vi "SAVEHWS.vi"(8 "error in (no error)":errorcluster, 9 "Enable (Array)":bool[](array[boolean]), 10 "data":waveform(dbl)[](array[waveform]), 11 "Destination HWS File":path) -> (0 "error out":errorcluster)   [LabVIEW 2011, in "DaqPad_NI6009.lvclass"]
uses:
  DaqPad_NI6009.lvclass
  niHWS Open File Permissions ID.ctl
panel:
  out "Waveform":waveform(dbl)(graph)
  out "Numeric":i32
  out "Array":string[](array[string])
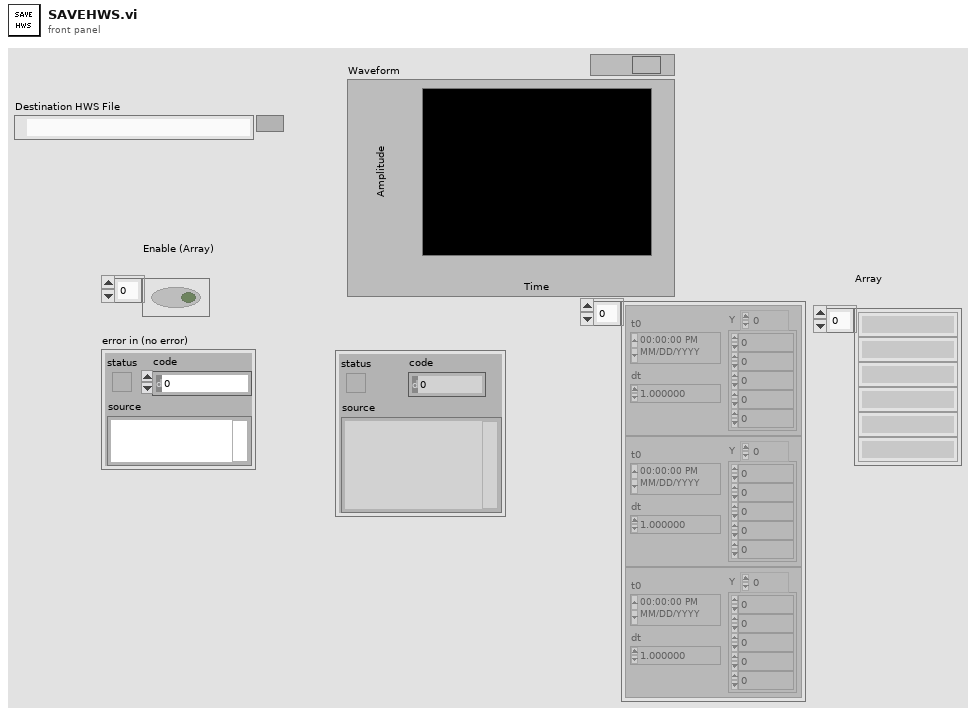
[diagram p1: front panel]
types:
  T1 = typedef "niHWS Open File Permissions ID.ctl" = enum32{"Read Only", "Read/Write Existing", "Read/Write/Create New", "Read/Write/Create New Always"}
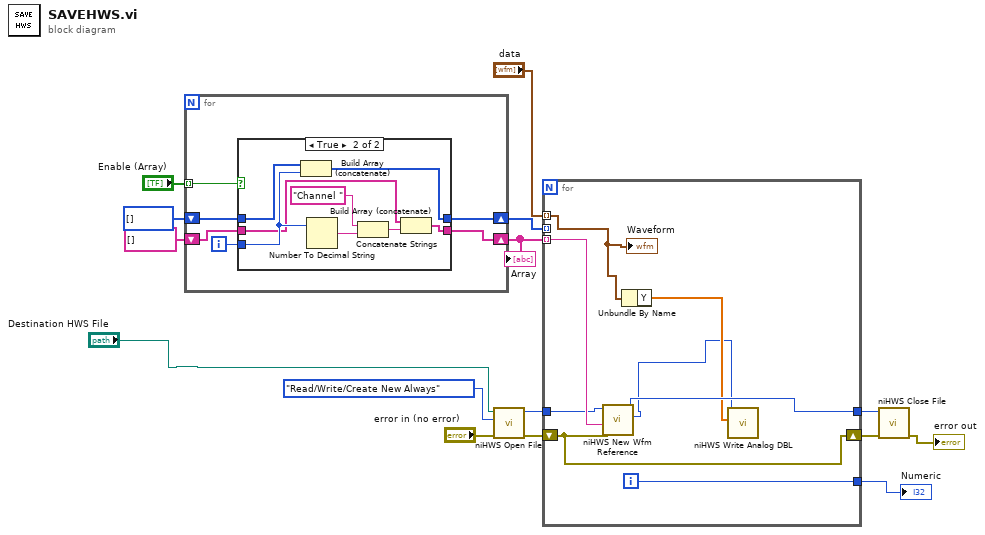
[diagram p0: block diagram]
diagram:
  n1 = for {
    tunnel: "Enable (Array)" -> [w21] mode=indexing
    shift-right: [w19] -> w14
    shift-left: i32[] [] -> [w18]
    shift-right: [w17] -> w15
    shift-left: string[] [] -> [w16]
    i -> [w20]
    n2 = case shown="True" w21 {
      tunnel: w20 -> [_ w26]
      tunnel: [w23 w31] -> w19
      tunnel: w18 -> [w23 w30]
      tunnel: [w22 w25] -> w17
      tunnel: w16 -> [w22 w24]
      frame False {
      }
      frame True {
        n3 = Build Array (concatenate)(w30, w26) -> (w31:i32[])
        n4 = Number To Decimal String(number=w26) -> (decimal integer string=w28:string)  [unwired: 1 in]
        n5 = Concatenate Strings("Channel ", w28) -> (w29:string)
        n6 = Build Array (concatenate)(w24, w29) -> (w25:string[])
      }
    }
  }
  "Array" <- w15
  n7 = call "niHWS Open File.vi"("error in (no error)"="error in (no error)", "permissions (0:read only)"=niHWS_Open_File_Permissions_ID."Read/Write/Create New Always" ("permissions"), "file path"="Destination HWS File") -> ("error out"=w8:errorcluster, "file handle"=w4:u32)  [unwired: 7 in]
  n8 = for {
    tunnel: w4 -> [w36]
    tunnel: "data" -> [w37] mode=indexing
    shift-right: [w35] -> w1
    shift-left: w8 -> [w35]
    tunnel: w14 -> [_] mode=indexing
    tunnel: w15 -> [w39] mode=indexing
    tunnel: [w38] -> w6
    tunnel: [w34] -> w3
    i -> [w38]
    n9 = call "niHWS New Wfm Reference.vi"("error in (no error)"=w35, "waveform name (empty)"=w39, "file handle in"=w36) -> ("waveform reference"=w32:u32, "file handle out"=w34:u32)  [unwired: 6 in, 1 out]
    n10 = Unbundle By Name(w37) -> ("Y"=w33:dbl[])
    n11 = call "niHWS Write Analog DBL.vi"("data"=w33, "waveform reference in"=w32) -> ()  [unwired: 8 in, 2 out]
    "Waveform" <- w37
  }
  "Numeric" <- w6
  n12 = call "niHWS Close File.vi"("error in (no error)"=w1, "file handle"=w3) -> ("error out"=→"error out":errorcluster)  [unwired: 9 in]
